vi "EPEC_Main.vi"() -> ()   [LabVIEW 2014]
panel:
  out "error out":errorcluster
  in  "error in":errorcluster
  in  "stop":bool
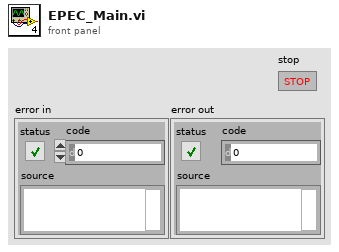
[diagram p1: front panel]
types:
  T1 = cluster{"PublicMessage":refnum<user-event>, "PrivateMessage":refnum<user-event>}
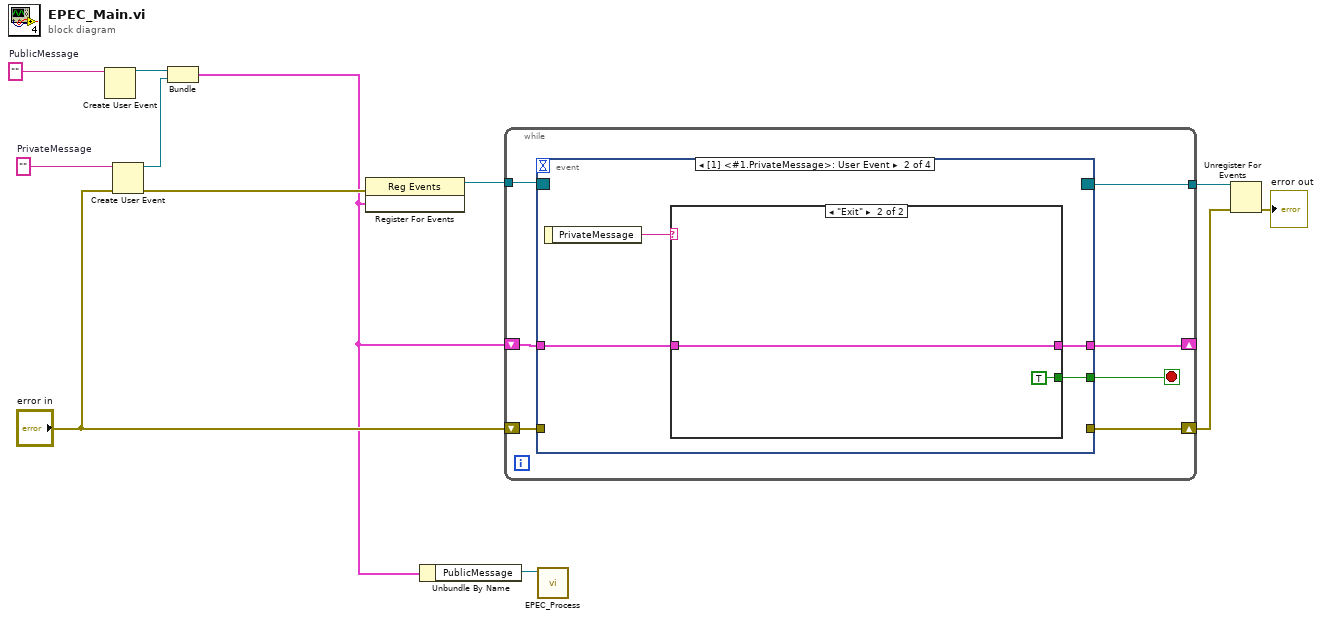
[diagram p0: block diagram]
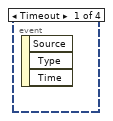
[diagram p2: hidden frame]
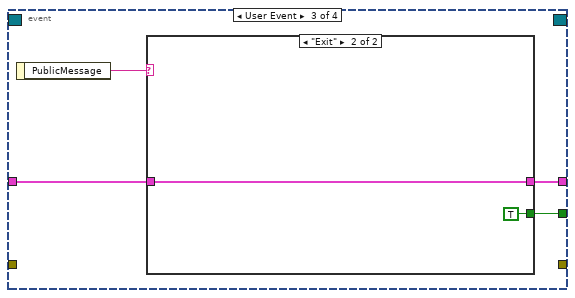
[diagram p4: hidden frame]
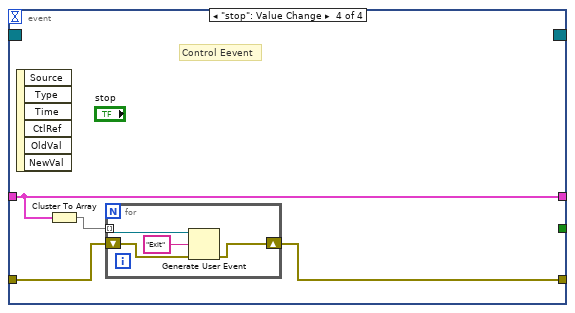
[diagram p6: hidden frame]
diagram:
  w5 = ""  # PublicMessage
  w10 = ""  # PrivateMessage
  n1 = Create User Event(user event datatype=w5) -> (user event=w4:refnum<user-event>)  [unwired: 1 in, 1 out]
  n2 = Create User Event(user event datatype=w10, error in="error in") -> (user event=w1:refnum<user-event>, error out=w11:errorcluster)
  n3 = Bundle("PublicMessage"=w4, "PrivateMessage"=w1) -> (w2:T1)  [unwired: 1 in]
  n4 = register-events(error in=w11, w2) -> (reference out=w12:refnum<event-registration>)  [unwired: 1 in, 1 out]
  n5 = Unbundle By Name(w2) -> ("PublicMessage"=w3:refnum<user-event>)
  n6 = while {
    tunnel: w12 -> [w19]
    shift-right: [w17] -> _
    shift-left: w2 -> [w18]
    shift-right: [w14] -> w8
    shift-left: "error in" -> [w15]
    tunnel: [w13] -> w9
    stop <- w16 stop-if-true
    n7 = event shown="[1] <#1.PrivateMessage>: User Event" {
      selector: w19 -> [_ _ _ _]
      dyn-events: [_ _ _ _] -> w13
      timeout: _ -> [_ _ _ _]
      tunnel: w18 -> [_ w21 w28 w37]
      tunnel: [_ w20 w27 w37] -> w17
      tunnel: [_ w23 w30 _] -> w16
      tunnel: w15 -> [_ _ _ w36]
      tunnel: [_ _ _ w35] -> w14
      event Timeout {
        n8 = event-data() -> ()  [unwired: 1 in, 3 out]
      }
      event User Event {
        n9 = event-data() -> ("PrivateMessage"=w22:string)  [unwired: 1 in]
        n10 = case shown="\"Exit\"" w22 {
          tunnel: [_ TRUE] -> w23
          tunnel: w21 -> [w24 w25]
          tunnel: [w24 w25] -> w20
          frame "False", Default {
          }
          frame "Exit" {
          }
        }
      }
      event User Event {
        n11 = event-data() -> ("PublicMessage"=w29:string)  [unwired: 1 in]
        n12 = case shown="\"Exit\"" w29 {
          tunnel: [_ TRUE] -> w30
          tunnel: w28 -> [w31 w32]
          tunnel: [w31 w32] -> w27
          frame "False", Default {
          }
          frame "Exit" {
          }
        }
      }
      event "stop": Value Change {
        # "Control Eevent"
        n13 = event-data() -> ()  [unwired: 1 in, 6 out]
        n14 = Cluster To Array(cluster=w37) -> (array=w34:refnum<user-event>[])
        n15 = for {
          tunnel: w34 -> [w38] mode=indexing
          shift-right: [w39] -> w35
          shift-left: w36 -> [w40]
          n16 = Generate User Event(user event=w38, event data cluster="Exit", error in=w40) -> (error out=w39:errorcluster)  [unwired: 1 in, 1 out]
        }
      }
    }
  }
  n17 = call "EPEC_Process.vi"("PublicMessage"=w3) -> ()  [unwired: 10 in, 1 out]
  n18 = Unregister For Events(event registration refnum=w9, error in=w8) -> (error out=→"error out":errorcluster)
